vi "GetLog.vi"(8 "Error in (no error)":errorcluster, 11 "LogWriterMock in":refnum<class "LogWriterMock.lvclass">) -> (0 "Error out":errorcluster, 2 "Array log out":T1[](array[typedef]) {"Priority" items=["EMERGENCY", "ALERT", "CRITICAL", "ERROR", "WARNING", "NOTICE", "INFO", "DEBUG"]}, 3 "LogWriterMock out":refnum<class "LogWriterMock.lvclass">)   [LabVIEW 2011, in "LogWriterMock.lvclass"]
uses:
  LogWriterMock.lvclass
  Log/LogCluster.ctl
  Log/PrioritiesRing.ctl
  LogWriterMock.lvclass/LogWriterMock.ctl
  Log/Log.lvclass
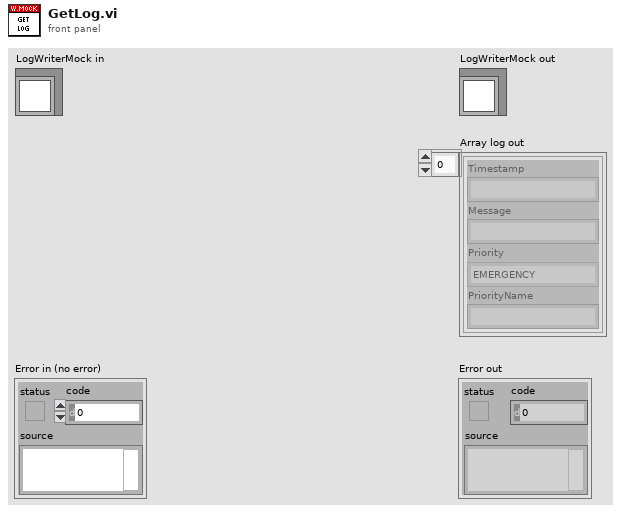
[diagram p1: front panel]
types:
  T1 = typedef "Log.lvclass/LogCluster.ctl" = cluster{"Timestamp":string, "Message":string, "Priority":T2, "PriorityName":string}
  T2 = typedef "Log.lvclass/PrioritiesRing.ctl" = u32
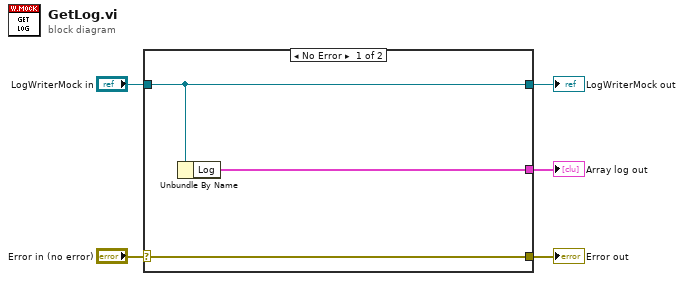
[diagram p0: block diagram]
diagram:
  n1 = case shown="No Error" "Error in (no error)" {
    selector: "Error in (no error)" -> [w8 w9]
    tunnel: [w8 w9] -> w4
    tunnel: [w7 w10] -> w2
    tunnel: "LogWriterMock in" -> [w7 w10]
    tunnel: [w6 _] -> w1
    frame No Error {
      n2 = Unbundle By Name(w7) -> ("Log"=w6:T1[])
    }
    frame Error {
    }
  }
  "Error out" <- w4
  "LogWriterMock out" <- w2
  "Array log out" <- w1
